vi "CANOpen Get Page Properties.vi"(8 "error in (no error)":errorcluster, 11 "This VI":refnum<vi>) -> (0 "error out":errorcluster, 3 "Settings":variant)   [LabVIEW 2021, in "CANOpen Addon System Explorer.lvlib"]
uses:
  CANOpen Addon System Explorer.lvlib
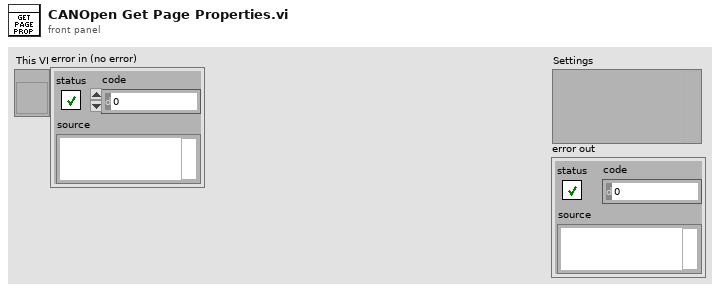
[diagram p1: front panel]
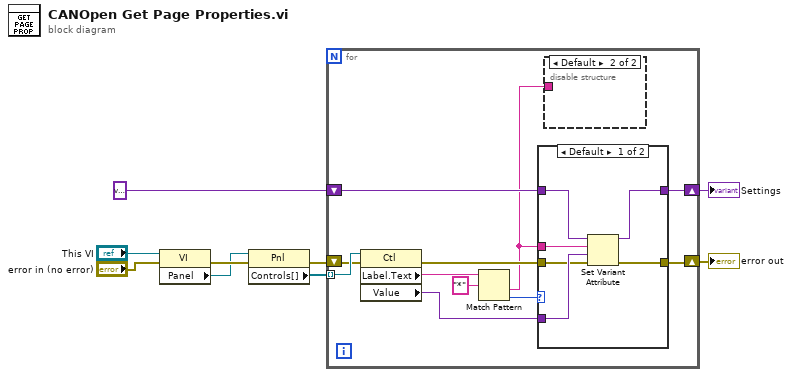
[diagram p0: block diagram]
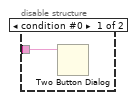
[diagram p2: hidden frame]
diagram:
  n1 = property class="VI"(reference="This VI", error in="error in (no error)") -> (error out=w7:errorcluster, "Panel"=w6:refnum<vi>)  [unwired: 1 out]
  n2 = property class="Pnl"(reference=w6, error in=w7) -> (error out=w4:errorcluster, "Controls[]"=w5:refnum<vi>[])  [unwired: 1 out]
  n3 = for {
    tunnel: w5 -> [w20] mode=indexing
    shift-right: [w12] -> w2
    shift-left: variant ("variant") -> [w15]
    shift-right: [w11] -> w1
    shift-left: w4 -> [w19]
    n4 = property class="Ctl"(reference=w20, error in=w19) -> (error out=w13:errorcluster, "Label.Text"=w18:string, "Value"=w14:variant)  [unwired: 1 out]
    n5 = Match Pattern(string=w18, regular expression="*") -> (after substring=w10:string, offset past match=w16:i32)  [unwired: 1 in, 2 out]
    n6 = case shown="Default" w16 {
      tunnel: w10 -> [w26 _]
      tunnel: w15 -> [w27 w29]
      tunnel: w14 -> [w25 _]
      tunnel: w13 -> [w24 w28]
      tunnel: [w23 w29] -> w12
      tunnel: [w22 w28] -> w11
      frame Default {
        n7 = Set Variant Attribute(Variant=w27, name=w26, value=w25, error in=w24) -> (Variant out=w23:variant, error out=w22:errorcluster)  [unwired: 1 out]
      }
      frame -1 {
      }
    }
    n8 = disable-structure shown="Default" {
      disable-tunnel: w10 -> [w21 _]
      frame condition #0 {
        n9 = Two Button Dialog(message=w21) -> ()  [unwired: 2 in, 1 out]
      }
      frame condition #1 (active) {
      }
    }
  }
  "Settings" <- w2
  "error out" <- w1
